vi "Read from Connection.vi"(8 "error in (no error)":errorcluster, 10 "Connection":refnum<class "IConnection.lvclass">, 11 "BasicNetworkProtocl in":refnum<class "BasicNetworkProtocol.lvclass">) -> (0 "error out":errorcluster, 2 "Data Read":string, 3 "BasicNetworkProtocl out":refnum<class "BasicNetworkProtocol.lvclass">)   [LabVIEW 2017, in "Network Logger Examples.lvlib" / "BasicNetworkProtocol.lvclass"]
uses:
  <vilib>/gpm_packages/@cs/event-logger/Examples/Examples/BasicNetworkProtocol/BasicNetworkProtocol.lvclass
  <vilib>/gpm_packages/@cs/Network-Sink/Source/Network Interface/IConnection/IConnection.lvclass
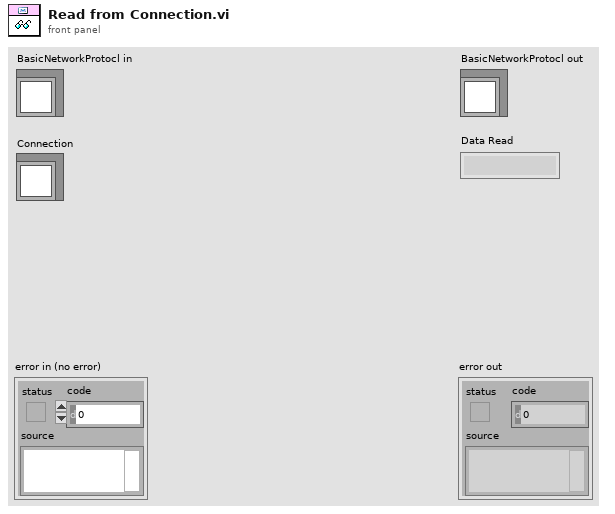
[diagram p1: front panel]
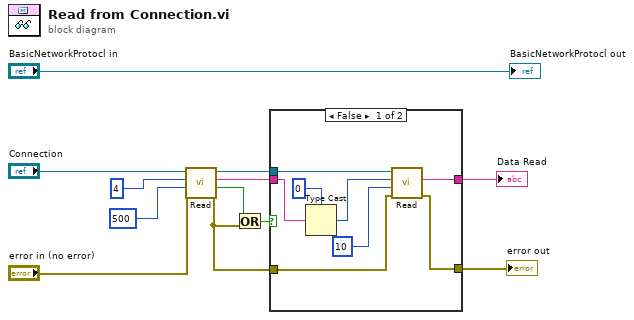
[diagram p0: block diagram]
diagram:
  n1 = call-dynamic "Read.vi"("error in (no error)"="error in (no error)", "Timeout (ms)"=500, "Bytes to Read"=4, "IConnection in"="Connection") -> ("error out"=w9:errorcluster, "TimeOut?"=w8:bool, "Data"=w7:string, "IConnection out"=w6:refnum<class "IConnection.lvclass">)  [unwired: 4 in]
  n2 = Or(x=w8, y=w9) -> (x .or. y?=w10:bool)
  n3 = case shown="False" w10 {
    tunnel: w9 -> [w16 w21]
    tunnel: w7 -> [w19 _]
    tunnel: w6 -> [w20 _]
    tunnel: [w14 w21] -> w2
    tunnel: [w13 _] -> w3
    frame False {
      n4 = Type Cast(type=0 ("Bytes to Read"), x=w19) -> (*(type *) &x=w17:i32)
      n5 = call-dynamic "Read.vi"("error in (no error)"=w16, "Timeout (ms)"=10, "Bytes to Read"=w17, "IConnection in"=w20) -> ("error out"=w14:errorcluster, "Data"=w13:string)  [unwired: 4 in, 2 out]
    }
    frame True {
    }
  }
  "error out" <- w2
  "Data Read" <- w3
  "BasicNetworkProtocl out" <- "BasicNetworkProtocl in"
